vi "Wiggle out from limit.vi"(6 "Steps":i64=100, 8 "error in (no error)":errorcluster, 9 "Retries":i32=5, 10 "Axis Number":i32, 11 "Agilis in":T1) -> (0 "error out":errorcluster, 3 "Agilis out":T1)   [LabVIEW 2016, in "Drivers.lvlib" / "Agilis.lvlib"]
uses:
  Agilis.lvlib
  AgilisCmdLib Refnum.ctl
  D:/Trace Grabber/Drivers/Agilis/AgilisCmdLib.dll
  AgilisCmdLib.dll
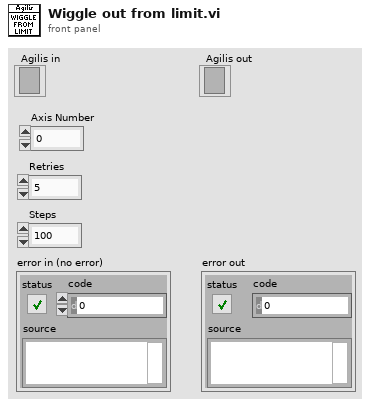
[diagram p1: front panel]
types:
  T1 = typedef "Drivers.lvlib/Agilis.lvlib/AgilisCmdLib Refnum.ctl" = refnum<k24>
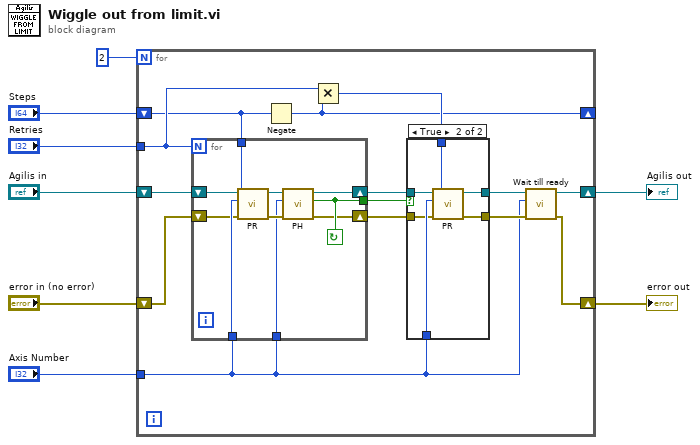
[diagram p0: block diagram]
diagram:
  n1 = for {
    N: 2 -> [_]
    tunnel: "Axis Number" -> [w9]
    tunnel: "Retries" -> [w19]
    shift-right: [w10] -> w7
    shift-left: "error in (no error)" -> [w14]
    shift-right: [w12] -> w1
    shift-left: "Agilis in" -> [w15]
    shift-right: [w16] -> _
    shift-left: "Steps" -> [w18]
    n2 = for {
      N: w19 -> [_]
      tunnel: w9 -> [w35]
      shift-right: [w38] -> w22
      shift-left: w15 -> [w31]
      tunnel: w18 -> [w37]
      tunnel: [w36] -> w21
      tunnel: w9 -> [w34]
      shift-right: [w33] -> w20
      shift-left: w14 -> [w32]
      stop <- w36 continue-if-true
      n3 = call "PR.vi"("error in (no error)"=w32, "Target Position"=w37, "Axis Number"=w35, "Agilis in"=w31) -> ("error out"=w40:errorcluster, "Agilis out"=w39:T1)  [unwired: 6 in]
      n4 = call "PH.vi"("error in (no error)"=w40, "Axis Number"=w34, "Agilis in"=w39) -> ("error out"=w33:errorcluster, "Triggered?"=w36:bool, "Agilis out"=w38:T1)  [unwired: 5 in, 1 out]
    }
    n5 = Negate(x=w18) -> (-x=w16:i64)
    n6 = Multiply(x=w19, y=w16) -> (x*y=w17:i64)
    n7 = case shown="True" w21 {
      tunnel: w22 -> [w24 w30]
      tunnel: [w24 w29] -> w13
      tunnel: w9 -> [_ w28]
      tunnel: w20 -> [w23 w27]
      tunnel: [w23 w26] -> w11
      tunnel: w17 -> [_ w25]
      frame False {
      }
      frame True {
        n8 = call "PR.vi"("error in (no error)"=w27, "Target Position"=w25, "Axis Number"=w28, "Agilis in"=w30) -> ("error out"=w26:errorcluster, "Agilis out"=w29:T1)  [unwired: 6 in]
      }
    }
    n9 = call "Wait till ready.vi"("error in (no error)"=w11, "Axis Number"=w9, ".NET Refnum in"=w13) -> ("error out"=w10:errorcluster, ".NET Refnum out"=w12:T1)  [unwired: 7 in]
  }
  "error out" <- w7
  "Agilis out" <- w1
